vi "uMsg_Delayed Daemon.vi"(11 "uMsg_Delayed in":refnum<class "uMsg_Delayed.lvclass">) -> ()   [LabVIEW 2021, in "uFramework.lvlib" / "uMsg_Delayed.lvclass"]
uses:
  uMsg_Delayed.lvclass
  uMsg_Delayed.lvclass/uMsg_Delayed.ctl
  uMsg/uMsg.lvclass/uMsg.ctl
  uMsg/uMsg Update Timestamp.vi
  uTransport/uTransport.lvclass
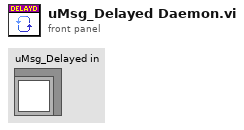
[diagram p1: front panel]
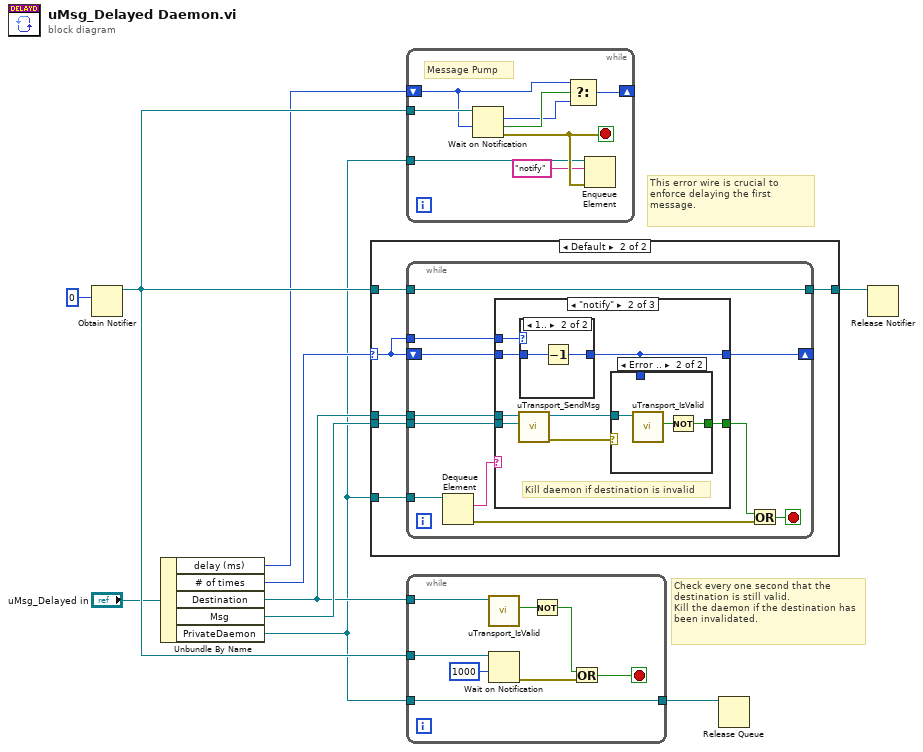
[diagram p0: block diagram]
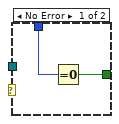
[diagram p5: hidden frame]
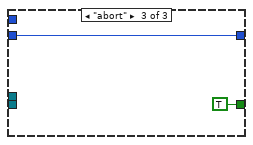
[diagram p6: hidden frame]
diagram:
  # "This error wire is crucial to enforce delaying the first message."
  # "Check every one second that the destination is still valid.\nKill the daemon if the destination has been invalidated."
  n1 = Obtain Notifier(notification data type=0) -> (notifier out=w8:refnum<notifier>)  [unwired: 3 in, 2 out]
  n2 = Unbundle By Name("uMsg_Delayed in") -> ("delay (ms)"=w5:i32, "# of times"=w4:i32, "Destination"=w2:refnum<class "uTransport.lvclass">, "Msg"=w3:refnum<class "uMsg.lvclass">, "PrivateDaemon"=w1:refnum<queue>)
  n3 = case shown="Default" w4 {
    selector: w4 -> [_ w13]
    tunnel: [w11 w17] -> w9
    tunnel: w8 -> [w11 w16]
    tunnel: w1 -> [_ w15]
    tunnel: w3 -> [_ w14]
    tunnel: w2 -> [_ w12]
    frame 0 {
    }
    frame Default {
      n4 = while {
        tunnel: w15 -> [w28]
        tunnel: w16 -> [w26]
        tunnel: [w26] -> w17
        tunnel: w14 -> [w25]
        shift-right: [w21] -> _
        shift-left: w13 -> [w24]
        tunnel: w13 -> [w22]
        tunnel: w12 -> [w23]
        stop <- w27 stop-if-true
        n5 = Dequeue Element(queue=w28) -> (element=w19:string, error out=w18:errorcluster)  [unwired: 2 in, 2 out]
        n6 = case shown="\"notify\"" w19 {
          tunnel: [_ w35 TRUE] -> w20
          tunnel: w25 -> [_ w34 _]
          tunnel: w24 -> [w29 w32 w47]
          tunnel: [w29 w30 w47] -> w21
          tunnel: w23 -> [_ w33 _]
          tunnel: w22 -> [_ w31 _]
          frame Default {
          }
          frame "notify" {
            # "Kill daemon if destination is invalid"
            n7 = call "uTransport_SendMsg.vi"("Msg"=w34, "uTransport in"=w33) -> ("error out"=w37:errorcluster, "uTransport out"=w36:refnum<class "uTransport.lvclass">)  [unwired: 8 in]
            n8 = case shown="1.." w31 {
              tunnel: [w38 w40] -> w30
              tunnel: w32 -> [w38 w39]
              frame ..0 {
              }
              frame 1.. {
                n9 = Decrement(x=w39) -> (x-1=w40:i32)
              }
            }
            n10 = case shown="Error .." w37 {
              tunnel: w36 -> [_ w45]
              tunnel: [w42 w43] -> w35
              tunnel: w30 -> [w41 _]
              frame No Error {
                n11 = Equal To 0?(x=w41) -> (x = 0?=w42:bool)
              }
              frame Error {
                n12 = call-dynamic "uTransport_IsValid.vi"("uTransport in"=w45) -> ("IsValid?"=w44:bool)  [unwired: 8 in, 2 out]
                n13 = Not(x=w44) -> (.not. x?=w43:bool)
              }
            }
          }
          frame "abort" {
          }
        }
        n14 = Or(x=w20, y=w18) -> (x .or. y?=w27:bool)
      }
    }
  }
  n15 = while {
    tunnel: w8 -> [w54]
    tunnel: w1 -> [w53]
    shift-right: [w50] -> _
    shift-left: w5 -> [w51]
    stop <- w55 stop-if-true
    # "Message Pump"
    n16 = Wait on Notification(notifier=w54, timeout in ms (-1)=w51) -> (notification=w49:i32, timed out?=w52:bool, error out=w55:errorcluster)  [unwired: 2 in, 1 out]
    n17 = Select(t=w51, s=w52, f=w49) -> (s? t:f=w50:i32)
    n18 = Enqueue Element(queue=w53, element="notify" ("CMD"), error in (no error)=w55) -> ()  [unwired: 1 in, 3 out]
  }
  n19 = while {
    tunnel: w1 -> [w63]
    tunnel: [w63] -> w10
    tunnel: w8 -> [w58]
    tunnel: w2 -> [w56]
    stop <- w61 stop-if-true
    n20 = call-dynamic "uTransport_IsValid.vi"("uTransport in"=w56) -> ("IsValid?"=w60:bool)  [unwired: 8 in, 2 out]
    n21 = Wait on Notification(notifier=w58, timeout in ms (-1)=1000) -> (error out=w62:errorcluster)  [unwired: 2 in, 3 out]
    n22 = Not(x=w60) -> (.not. x?=w59:bool)
    n23 = Or(x=w59, y=w62) -> (x .or. y?=w61:bool)
  }
  n24 = Release Queue(queue=w10) -> ()  [unwired: 2 in, 3 out]
  n25 = Release Notifier(notifier=w9) -> ()  [unwired: 2 in, 3 out]
